vi "TRANCON-HARDWARE-SERVER.vi"() -> ()   [LabVIEW 2015]
doc: "MAIN vi for TRANCON project"
uses:
  dependecies/XControls/StartButton/StartButton.xctl
  <vilib>/NI/STM/Connection Manager/TCP/TCP Connection Method.ctl
  Classes/Control/Control-Server/Control-Server.lvclass
  dependecies/ControlsVIs/Clusters-def/DEFs_SERVER_buttons_refs.ctl
  Classes/Control/Control-Server/Control-Server.lvclass/Control-Server.ctl
  Classes/GeneralFunctionality/GeneralFunctionality.lvclass/GeneralFunctionality.ctl
  <vilib>/Platform/TimedLoop/XDataNode/timing_clust.ctl
  <vilib>/Platform/TimedLoop/XDataNode/nitl_modes.ctl
  <vilib>/Platform/TimedLoop/XDataNode/wakeup.ctl
  dependecies/ControlsVIs/Clusters-def/Message types.ctl
  dependecies/ControlsVIs/Clusters-def/SERVER-Commands.ctl
  Classes/Config/config_names_def.ctl
  <vilib>/NI/STM/TCP/Write Meta Data (TCP Ref).vi
  <vilib>/NI/STM/TCP/Write Meta Data (TCP Clst).vi
  <vilib>/Platform/TimedLoop/XDataNode/XDataNode.xnode
  Classes/Config/Config.lvclass
  <vilib>/NI/STM/NI STM.lvlib
  <vilib>/Platform/TimedLoop/XDataNode/XDNodeRunTimeDep.lvlib
  Classes/Message/Message.lvclass
  Classes/GeneralFunctionality/GeneralFunctionality.lvclass
panel:
  in  "DB Set":bool
  in  "DB connect":bool
  in  "OSc Set":bool
  in  "Oscilloscope connect":bool
  in  "DAQmx Set":bool
  in  "DAQmx connect":bool
  in  "DET Set":bool
  in  "Detector connect":bool
  in  "DL Set":bool
  in  "DL connect":bool
  in  "All connect":bool
  in  "Pump connect":bool
  out "# clients":i32
  out "stop":bool
  in  "StartButton":bool(xcontrol)
  out "error out":cluster{bool, i32, "source":string} {"?" format="%f"}
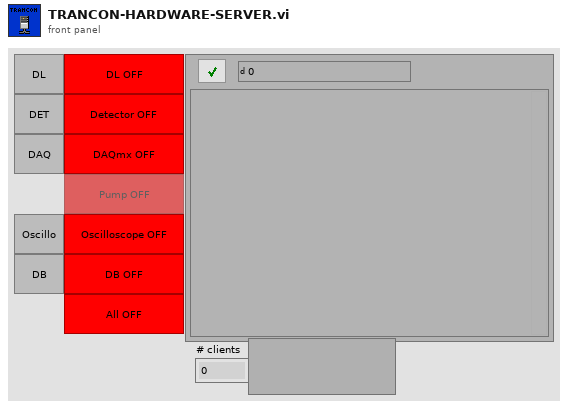
[diagram p1: front panel]
types:
  T1 = typedef "Control-Server.lvclass/DEFs_SERVER_buttons_refs.ctl" = cluster{"DL connect":refnum<vi>, "Detector connect":refnum<vi>, "DAQmx connect":refnum<vi>, "OSc connect":refnum<vi>, "DB connect":refnum<vi>, "All connect":refnum<vi>}
  T2 = typedef "NI STM.lvlib/TCP Connection Method.ctl" = enum16{"Initialize", "Add Connection", "Set Properties", "Get Connection(s)", "Remove Connection", "Remove All Connections", "Get Connection Count"}
  T3 = typedef "NI STM.lvlib/TCP Connection Info.ctl" = cluster{"connection ID":refnum<k5>, "meta data":T4[]}
  T4 = typedef "NI STM.lvlib/MetaDataElement.ctl" = string
  T5 = typedef "XDNodeRunTimeDep.lvlib/timing_clust.ctl" = cluster{"Expected End [f-1]":u64, "Actual End [f-1]":u64, "Finished Late? [f-1]":bool, "Expected End [i-1]":u64, "Actual End [i-1]":u64, "Finished Late? [i-1]":bool, "Expected Start [i]":u64, "Actual Start [i]":u64, "Expected Start [f]":u64, "Actual Start [f]":u64, "Source Name":string, "Structure Name":string, "Period":i64, "Deadline":i64, "Offset":i64, "Start":i64, "Priority":i32, "Timeout":i32, "Mode":T6, "Wakeup Reason":T7, "Error":errorcluster, "Source Type":string, "Secondary Source Type":string, "Global End Time":u64, "Global Start Time":u64, "Frame Duration":u64, "Iteration Duration":u64, "Assigned CPU":i32, "I/O Scan Engine Mode":u32}
  T6 = typedef "XDNodeRunTimeDep.lvlib/nitl_modes.ctl" = enum32{"No Change", "Process missed periods, maintain original phase", "Discard missed periods, maintain original phase", "Process missed periods, ignore original phase", "Discard missed periods, ignore original phase"}
  T7 = typedef "XDNodeRunTimeDep.lvlib/wakeup.ctl" = enum32{"Normal", "Aborted", "Asynchronous wakeup", "Timing source error", "Timed loop error", "Timeout"}
  T8 = typedef "Control-Server.lvclass/SERVER-Commands.ctl" = string
  T9 = typedef "Message types.ctl" = string
  T10 = typedef "Config.lvclass/config_names_def.ctl" = string
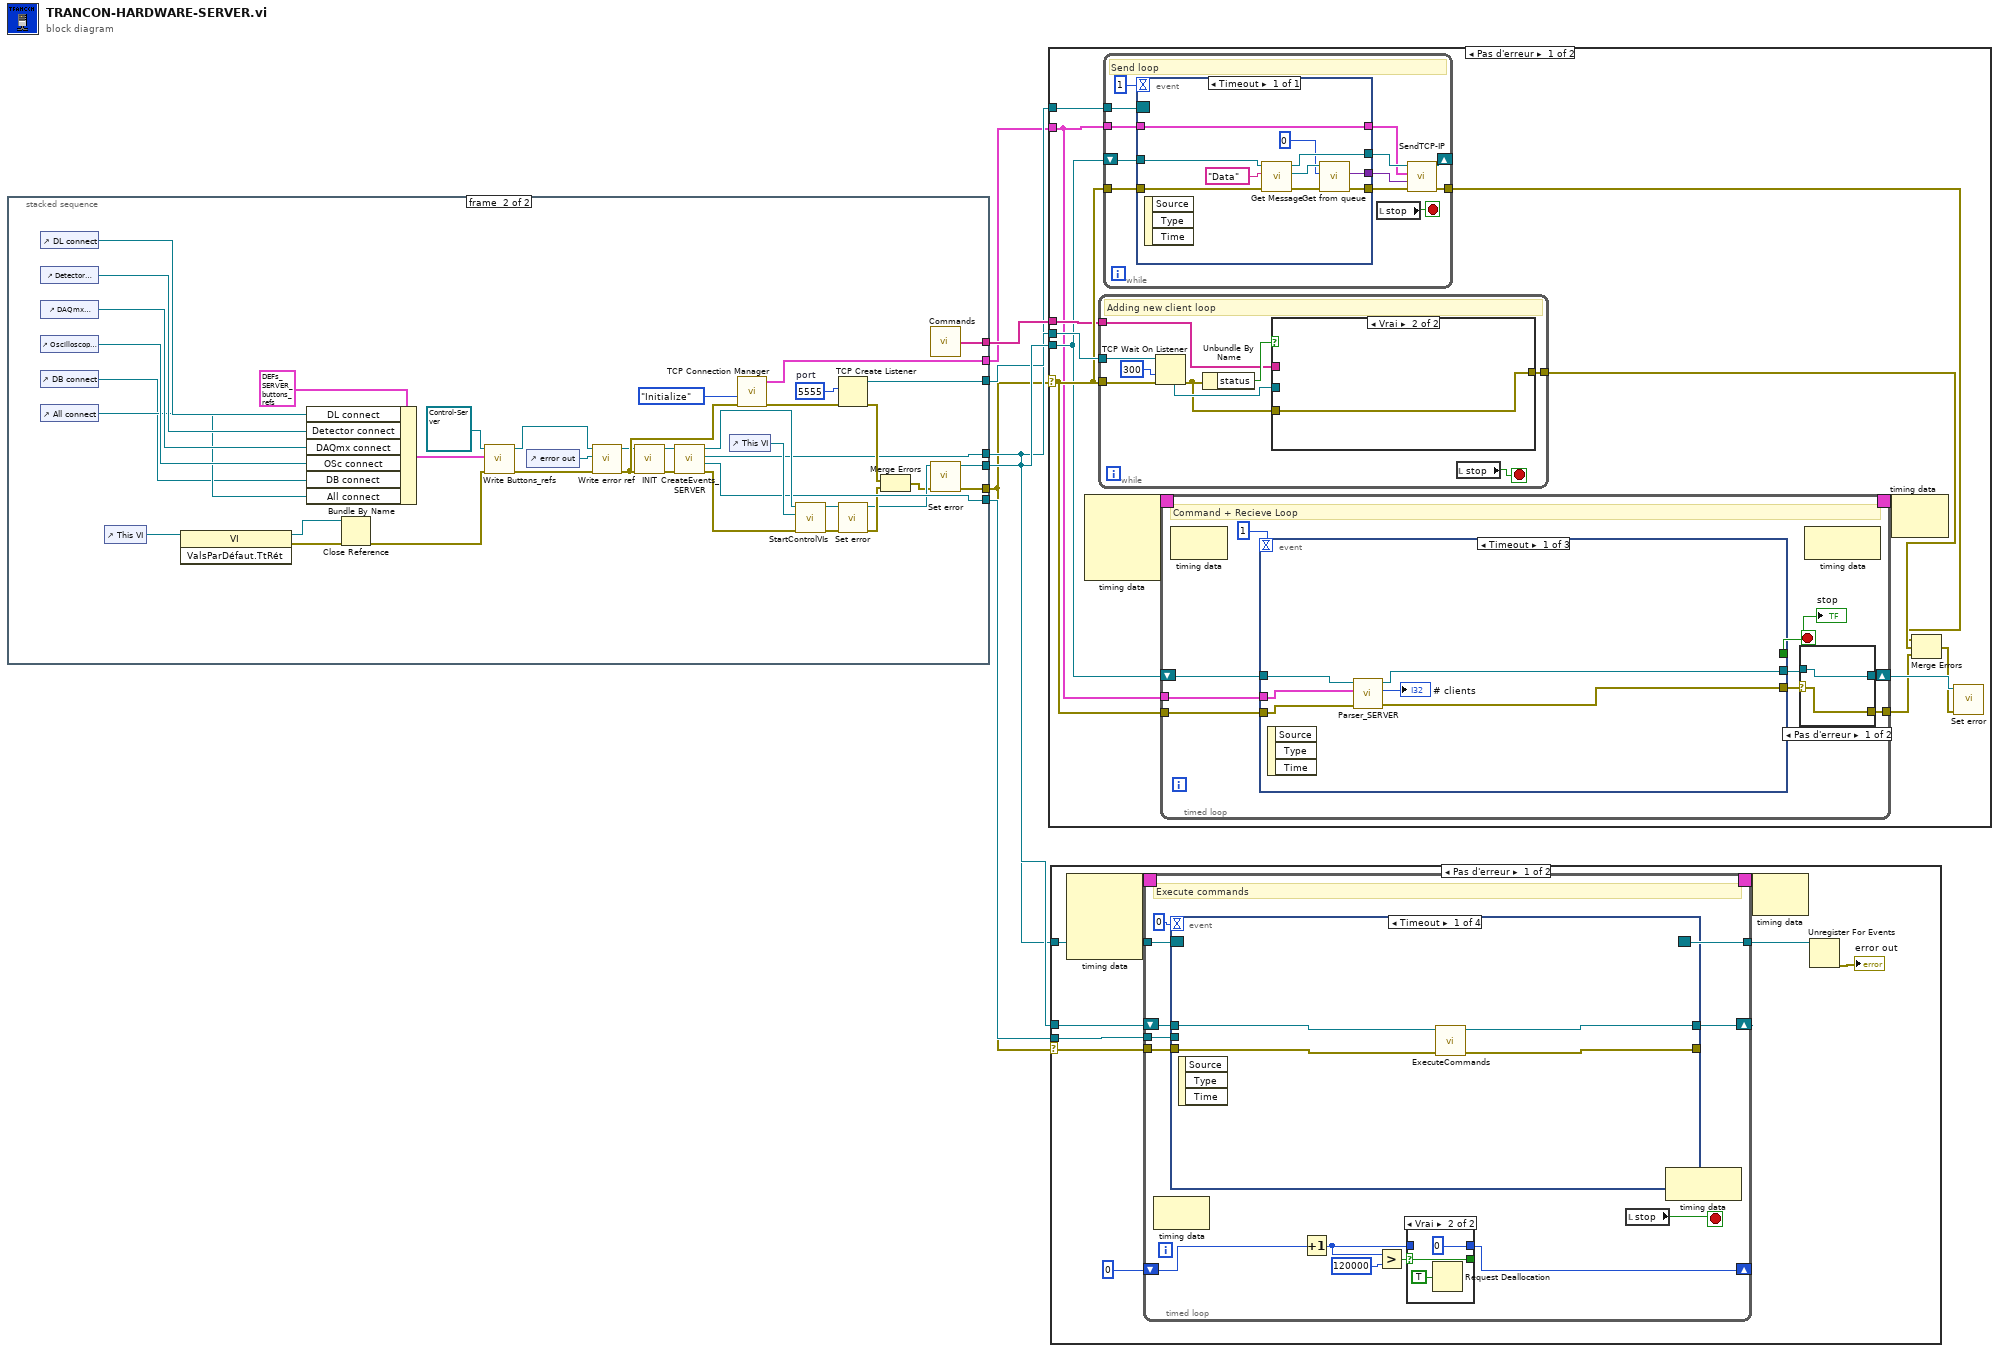
[diagram p0: block diagram]
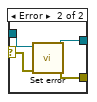
[diagram p2: hidden frame]
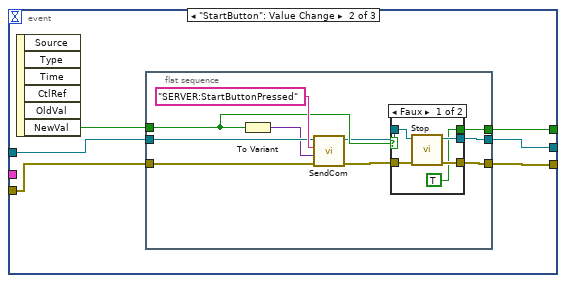
[diagram p3: hidden frame]
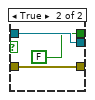
[diagram p4: hidden frame]
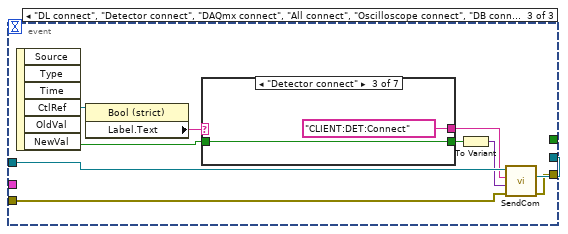
[diagram p5: hidden frame]
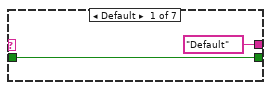
[diagram p6: hidden frame]
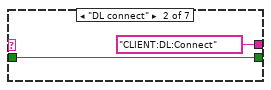
[diagram p7: hidden frame]
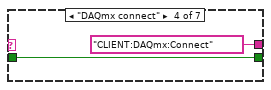
[diagram p8: hidden frame]
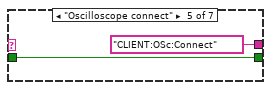
[diagram p9: hidden frame]
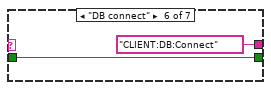
[diagram p10: hidden frame]
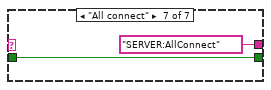
[diagram p11: hidden frame]
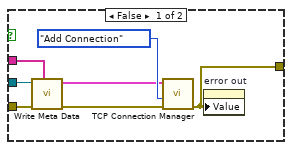
[diagram p12: hidden frame]
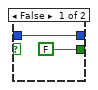
[diagram p14: hidden frame]
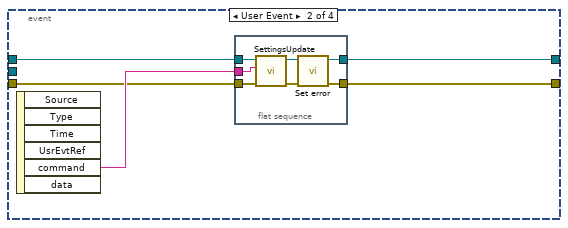
[diagram p15: hidden frame]
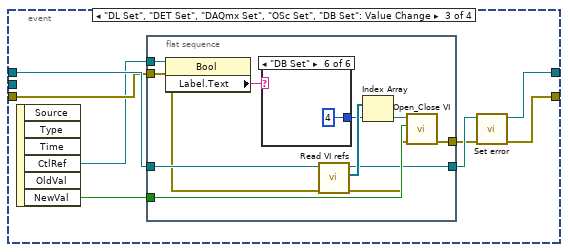
[diagram p16: hidden frame]
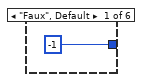
[diagram p17: hidden frame]
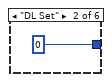
[diagram p18: hidden frame]
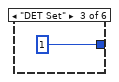
[diagram p19: hidden frame]
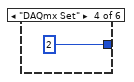
[diagram p20: hidden frame]
diagram:
  n1 = stacked-sequence {
    tunnel: [_ w24] -> w6
    tunnel: [_ w21] -> w3
    tunnel: [_ w42] -> w7
    tunnel: [_ w20] -> w5
    tunnel: [_ w35] -> w4
    tunnel: [_ w34] -> w1
    tunnel: [_ w23] -> w2
    frame #0 {
      n2 = flat-sequence {
        frame #0 {
        }
      }
    }
    frame #1 {
      w38 = u16 5555  # port
      n3 = control-ref of="DL connect"() -> (w15:refnum<vi>)
      n4 = control-ref of="Detector connect"() -> (w13:refnum<vi>)
      n5 = control-ref of="DAQmx connect"() -> (w12:refnum<vi>)
      n6 = control-ref of="Oscilloscope connect"() -> (w11:refnum<vi>)
      n7 = control-ref of="DB connect"() -> (w9:refnum<vi>)
      n8 = control-ref of="All connect"() -> (w10:refnum<vi>)
      n9 = control-ref of="This VI"() -> (w41:refnum<vi>)
      n10 = invoke class="VI" method="ValsParDéfaut.TtRét"(reference=w41) -> (reference out=w40:refnum<vi>, error out=w39:errorcluster)  [unwired: 2 in, 1 out]
      n11 = Bundle By Name(cluster=T1 {"DL connect"=refnum, "Detector connect"=refnum, "DAQmx connect"=refnum, "OSc connect"=refnum, "DB connect"=refnum, "All connect"=refnum} ("input cluster"), "DL connect"=w15, "Detector connect"=w13, "DAQmx connect"=w12, "OSc connect"=w11, "DB connect"=w9, "All connect"=w10) -> (w8:T1)
      n12 = Close Reference(reference=w40, error in (no error)=w39) -> (error out=w19:errorcluster)
      n13 = call "Write Buttons_refs.vi"("error in (no error)"=w19, "input cluster"=w8, "Control-Server in"=refnum<class "Control-Server.lvclass"> refnum) -> ("error out"=w18:errorcluster, "Control-Server out"=w17:refnum<class "Control-Server.lvclass">)  [unwired: 7 in]
      n14 = control-ref of="error out"() -> (w33:refnum<vi>)
      n15 = call "Write error ref.vi"("error in (no error)"=w18, "error"=w33, "GeneralFunctionality in"=w17) -> ("error out"=w29:errorcluster, "GeneralFunctionality out"=w28:refnum<class "Control-Server.lvclass">)  [unwired: 7 in]
      n16 = call-dynamic "INIT.vi"("error in (no error)"=w29, "Control-Server in"=w28) -> ("error out"=w32:errorcluster, "Control-Server out"=w45:refnum<class "Control-Server.lvclass">)  [unwired: 8 in]
      n17 = call "CreateEvents_SERVER.vi"("error in (no error)"=w32, "Control class"=w45) -> ("error out"=w43:errorcluster, "SettingsEventCom"=w42:refnum<user-event>, "Event Registration Refnum"=w21:refnum<event-registration>, "Control class out"=w44:refnum<class "Control-Server.lvclass">)  [unwired: 6 in]
      n18 = control-ref of="This VI"() -> (w46:refnum<vi>)
      n19 = call <vilib>:"TCP Connection Manager.vi"("error in"=w29, "method"=TCP_Connection_Method."Initialize") -> ("error out"=w36:errorcluster, "connection out"=w34:T3)  [unwired: 4 in, 4 out]
      n20 = call "StartControlVIs.vi"("entrée d'erreur (pas d'erreur)"=w43, "This VI"=w46, "Control in"=w44) -> ("sortie d'erreur"=w30:errorcluster, "Control out"=w31:refnum<class "Control-Server.lvclass">)  [unwired: 7 in]
      n21 = TCP Create Listener(8:w36, 10:w38) -> (0:w26:errorcluster, 3:w35:refnum<k5>)  [unwired: 3 in, 1 out]
      n22 = call "Set error.vi"("error in (no error)"=w30, "Control-Server in"=w31) -> ("error out"=w27:errorcluster, "Control-Server out"=w25:refnum<class "Control-Server.lvclass">)  [unwired: 8 in]
      n23 = Merge Errors(w26, w27) -> (w22:errorcluster)
      n24 = call "Commands.vi"() -> ("Commands"=w20:T4[])
      n25 = call "Set error.vi"("error in (no error)"=w22, "Control-Server in"=w25) -> ("error out"=w23:errorcluster, "Control-Server out"=w24:refnum<class "Control-Server.lvclass">)  [unwired: 8 in]
    }
  }
  n26 = case shown="Pas d'erreur" w2 {
    selector: w2 -> [w58 _]
    tunnel: w6 -> [w56 _]
    tunnel: w4 -> [w59 _]
    tunnel: w5 -> [w57 _]
    tunnel: w1 -> [w51 _]
    tunnel: w3 -> [w55 _]
    frame No Error {
      n27 = node-c288() -> (w54:T5)  [unwired: 4 in]
      n28 = while "Listen loop.  Append new connections to a synchronized queue." {
        tunnel: w57 -> [w161]
        tunnel: w58 -> [w159]
        tunnel: w59 -> [w158]
        tunnel: [w156] -> w49
        stop <- w157 stop-if-true
        # "Adding new client loop"
        n29 = TCP Wait On Listener(8:w159, 9:300 ("timeout ms (wait forever: -1)"), 11:w158) -> (0:w160:errorcluster, 4:w163:refnum<k5>)  [unwired: 1 in, 3 out]
        n30 = Unbundle By Name(w160) -> ("status"=w162:bool)
        n31 = case shown="Vrai" w162 {
          tunnel: w163 -> [w170 _]
          tunnel: w161 -> [w165 _]
          tunnel: w160 -> [w168 w171]
          tunnel: [w164 w171] -> w156
          frame False {
            n32 = call-poly <vilib>:"Write Meta Data.vi"("meta data"=w165, "error in"=w168, "connection ID"=w170) -> ("error out"=w169:errorcluster, "connection info out"=w166:T3)  [unwired: 7 in]
            n33 = call <vilib>:"TCP Connection Manager.vi"("error in"=w169, "method"=TCP_Connection_Method."Add Connection", "connection in"=w166) -> ("error out"=w164:errorcluster)  [unwired: 3 in, 5 out]
            n34 = property on="error out" class="Clust (strict)"("Value"=w164) -> ()  [unwired: 2 in, 2 out]
          }
          frame True {
          }
        }
        n35 = local read "stop"() -> (w157:bool)
      }
      n36 = while {
        tunnel: w58 -> [w143]
        tunnel: [w137] -> w48
        tunnel: w51 -> [w142]
        shift-right: [w136] -> _
        shift-left: w56 -> [w144]
        tunnel: w55 -> [w140]
        stop <- w133 stop-if-true
        # "Send loop"
        n37 = event shown="[0] Timeout" {
          selector: w140 -> [_]
          dyn-events: _ -> [_]
          timeout: 1 -> [_]
          tunnel: w144 -> [w154]
          tunnel: w143 -> [w153]
          tunnel: w142 -> [w149]
          tunnel: [w152] -> w139
          tunnel: [w151] -> w138
          tunnel: [w150] -> w135
          tunnel: [w149] -> w134
          event Timeout {
            n38 = event-data() -> ()  [unwired: 1 in, 3 out]
            n39 = call "Get Message.vi"("error in (no error)"=w153, "Message type"=T9 "Data", "GeneralFunctionality en entrée"=w154) -> ("error out"=w147:errorcluster, "Message.lvclass"=w146:refnum<class "Message.lvclass">, "GeneralFunctionality en sortie"=w150:refnum<class "Control-Server.lvclass">)  [unwired: 6 in]
            n40 = call "Get from queue.vi"("error in (no error)"=w147, "timeout in ms (-1)"=0, "Message in"=w146) -> ("error out"=w151:errorcluster, "Data"=w152:variant)  [unwired: 5 in, 2 out]
          }
        }
        n41 = local read "stop"() -> (w133:bool)
        n42 = call "SendTCP-IP.vi"("error in (no error)"=w138, "Data"=w139, "connection in"=w134, "Control in"=w135) -> ("error out"=w137:errorcluster, "Control out"=w136:refnum<class "Control-Server.lvclass">)  [unwired: 6 in]
      }
      n43 = timed-loop {
        tunnel: w58 -> [w68]
        tunnel: w51 -> [w67]
        shift-right: [w61] -> w52
        shift-left: w56 -> [w65]
        timing: w54 -> [_]
        timing-out: [_] -> w53
        tunnel: [w63] -> w50
        stop <- w64 stop-if-true
        # "Command + Recieve Loop"
        n44 = node-c288() -> ()  [unwired: 1 in, 1 out]
        n45 = event shown="[0] Timeout" {
          selector: _ -> [_ _ _]
          dyn-events: _ -> [_ _ _]
          timeout: 1 -> [_ _ _]
          tunnel: w65 -> [w78 w87 w115]
          tunnel: w68 -> [w82 w86 w116]
          tunnel: [w80 w83 w107] -> w60
          tunnel: w67 -> [w79 _ _]
          tunnel: [w77 w84 w108] -> w62
          tunnel: [_ w85 _] -> w64
          event Timeout {
            n46 = event-data() -> ()  [unwired: 1 in, 3 out]
            n47 = call "Parser_SERVER.vi"("error in (no error)"=w82, "connection in"=w79, "Control in"=w78) -> ("error out"=w80:errorcluster, "# clients"=→"# clients":i32, "Control out"=w77:refnum<class "Control-Server.lvclass">)  [unwired: 6 in]
          }
          event "StartButton": Value Change {
            n48 = event-data() -> ("NewVal"=w88:bool)  [unwired: 1 in, 5 out]
            n49 = flat-sequence {
              tunnel: w88 -> [w94]
              tunnel: w87 -> [w97]
              tunnel: [w91] -> w84
              tunnel: [w90] -> w83
              tunnel: w86 -> [w96]
              tunnel: [w89] -> w85
              frame #0 {
                n50 = To Variant(anything=w94) -> (Variant=w95:variant)
                n51 = call "SendCom.vi"("error in (no error)"=w96, "data"=w95, "Command"="SERVER:StartButtonPressed", "Control in"=w97) -> ("error out"=w92:errorcluster, "Control out"=w93:refnum<class "Control-Server.lvclass">)  [unwired: 6 in]
                n52 = case shown="Faux" w94 {
                  tunnel: [w103 w106] -> w91
                  tunnel: [w102 w105] -> w90
                  tunnel: w93 -> [w100 w106]
                  tunnel: w92 -> [w101 w105]
                  tunnel: [TRUE FALSE] -> w89
                  frame False {
                    n53 = call-dynamic "Stop.vi"("error in (no error)"=w101, "Control in"=w100) -> ("error out"=w102:errorcluster, "Control out"=w103:refnum<class "Control-Server.lvclass">)  [unwired: 8 in]
                  }
                  frame True {
                  }
                }
              }
            }
          }
          event "DL connect", "Detector connect", "DAQmx connect", "All connect", "Oscilloscope connect", "DB connect": Value Change {
            n54 = event-data() -> ("CtlRef"=w114:refnum<vi>, "NewVal"=w111:bool)  [unwired: 1 in, 4 out]
            n55 = property class="Bool (strict)"(reference=w114) -> ("Label.Text"=w113:string)  [unwired: 1 in, 2 out]
            n56 = case shown="\"Detector connect\"" w113 {
              tunnel: [T8 "Default" ("Commands") T8 "CLIENT:DL:Connect" ("Commands") T8 "CLIENT:DET:Connect" ("Commands") T8 "CLIENT:DAQmx:Connect" ("Commands") T8 "CLIENT:OSc:Connect" ("Commands") T8 "CLIENT:DB:Connect" ("Commands") T8 "SERVER:AllConnect" ("Commands")] -> w112
              tunnel: w111 -> [w117 w119 w121 w123 w125 w127 w129]
              tunnel: [w117 w119 w121 w123 w125 w127 w129] -> w110
              frame Default {
              }
              frame "DL connect" {
              }
              frame "Detector connect" {
              }
              frame "DAQmx connect" {
              }
              frame "Oscilloscope connect" {
              }
              frame "DB connect" {
              }
              frame "All connect" {
              }
            }
            n57 = To Variant(anything=w110) -> (Variant=w109:variant)
            n58 = call "SendCom.vi"("error in (no error)"=w116, "data"=w109, "Command"=w112, "Control in"=w115) -> ("error out"=w107:errorcluster, "Control out"=w108:refnum<class "Control-Server.lvclass">)  [unwired: 6 in]
          }
        }
        "stop" <- w64
        n59 = case shown="Pas d'erreur" w60 {
          selector: w60 -> [w69 w71]
          tunnel: [w69 w74] -> w63
          tunnel: w62 -> [w70 w73]
          tunnel: [w70 w72] -> w61
          frame No Error {
          }
          frame Error {
            n60 = call "Set error.vi"("error in (no error)"=w71, "Control-Server in"=w73) -> ("error out"=w74:errorcluster, "Control-Server out"=w72:refnum<class "Control-Server.lvclass">)  [unwired: 8 in]
          }
        }
        n61 = node-c288() -> ()  [unwired: 1 in, 1 out]
      }
      n62 = node-c288(w53) -> ()  [unwired: 1 out]
      n63 = Merge Errors(w48, w49, w50) -> (w47:errorcluster)
      n64 = call "Set error.vi"("error in (no error)"=w47, "Control-Server in"=w52) -> ()  [unwired: 8 in, 2 out]
    }
    frame Error {
    }
  }
  n65 = case shown="Pas d'erreur" w2 {
    selector: w2 -> [w178 _]
    tunnel: w6 -> [w180 _]
    tunnel: w3 -> [w177 _]
    tunnel: w7 -> [w176 _]
    frame No Error {
      n66 = node-c288() -> (w175:T5)  [unwired: 4 in]
      n67 = timed-loop {
        shift-right: [w191] -> _
        shift-left: w180 -> [w192]
        tunnel: w178 -> [w193]
        tunnel: [w190] -> w179
        tunnel: w177 -> [w189]
        tunnel: w176 -> [w188]
        timing: w175 -> [_]
        timing-out: [_] -> w174
        shift-right: [w181] -> _
        shift-left: 0 -> [w182]
        stop <- w186 stop-if-true
        # "Execute commands"
        n68 = node-c288() -> ()  [unwired: 1 in, 1 out]
        n69 = event shown="[0] Timeout" {
          selector: w189 -> [_ _ _ _]
          dyn-events: [_ _ _ _] -> w190
          timeout: 0 -> [_ _ _ _]
          tunnel: [w201 w205 w219 w242] -> _
          tunnel: w193 -> [w203 w207 w223 w247]
          tunnel: w192 -> [w204 w208 w224 w244]
          tunnel: [w202 w206 w218 w243] -> w191
          tunnel: w188 -> [_ _ _ w246]
          event Timeout {
            n70 = event-data() -> ()  [unwired: 1 in, 3 out]
            n71 = call "ExecuteCommands.vi"("error in (no error)"=w203, "Control in"=w204) -> ("error out"=w201:errorcluster, "Control out"=w202:refnum<class "Control-Server.lvclass">)  [unwired: 8 in]
          }
          event User Event {
            n72 = event-data() -> ("command"=w209:string)  [unwired: 1 in, 5 out]
            n73 = flat-sequence {
              tunnel: w209 -> [w216]
              tunnel: w208 -> [w215]
              tunnel: w207 -> [w214]
              tunnel: [w212] -> w206
              tunnel: [w210] -> w205
              frame #0 {
                n74 = call "SettingsUpdate.vi"("error in (no error)"=w214, "Command"=w216, "Control in"=w215) -> ("error out"=w211:errorcluster, "Control out"=w213:refnum<class "Control-Server.lvclass">)  [unwired: 7 in]
                n75 = call "Set error.vi"("error in (no error)"=w211, "Control-Server in"=w213) -> ("error out"=w210:errorcluster, "Control-Server out"=w212:refnum<class "Control-Server.lvclass">)  [unwired: 8 in]
              }
            }
          }
          event "DL Set", "DET Set", "DAQmx Set", "OSc Set", "DB Set": Value Change {
            n76 = event-data() -> ("CtlRef"=w217:refnum<vi>, "NewVal"=w222:bool)  [unwired: 1 in, 4 out]
            n77 = flat-sequence {
              tunnel: [w230] -> w221
              tunnel: w224 -> [w233]
              tunnel: w223 -> [w226]
              tunnel: w222 -> [w235]
              tunnel: [w234] -> w220
              tunnel: w217 -> [w229]
              frame #0 {
                n78 = property class="Bool"(reference=w229) -> ("Label.Text"=w228:string)  [unwired: 1 in, 2 out]
                n79 = case shown="\"DB Set\"" w228 {
                  tunnel: [-1 0 1 2 3 4] -> w227
                  frame "Faux", Default {
                  }
                  frame "DL Set" {
                  }
                  frame "DET Set" {
                  }
                  frame "DAQmx Set" {
                  }
                  frame "OSc Set" {
                  }
                  frame "DB Set" {
                  }
                }
                n80 = call-dynamic "Read VI refs.vi"("error in (no error)"=w226, "Control in"=w233) -> ("error out"=w225:errorcluster, "VI refs"=w232:refnum<vi>[], "Control out"=w230:refnum<class "Control-Server.lvclass">)  [unwired: 7 in]
                n81 = Index Array(array=w232, index=w227) -> (element=w231:refnum<vi>)
                n82 = call "Open_Close VI.vi"("error in (no error)"=w225, "NewVal"=w235, "VI in"=w231) -> ("error out"=w234:errorcluster)  [unwired: 8 in]
              }
            }
            n83 = call "Set error.vi"("error in (no error)"=w220, "Control-Server in"=w221) -> ("error out"=w219:errorcluster, "Control-Server out"=w218:refnum<class "Control-Server.lvclass">)  [unwired: 8 in]
          }
          event Menu Selection (User) {
            n84 = event-data() -> ("ItemTag"=w248:string)  [unwired: 1 in, 6 out]
            n85 = flat-sequence {
              tunnel: w248 -> [w254]
              tunnel: w247 -> [w253]
              tunnel: [w252] -> w245
              tunnel: w244 -> [w251]
              tunnel: w246 -> [w249]
              frame #0 {
                n86 = case shown="\"Settings\"" w254 {
                  tunnel: w253 -> [w258 w263]
                  tunnel: [w261 w263] -> w252
                  tunnel: w251 -> [w260 _]
                  tunnel: TRUE ("stop? (T)") -> [_ w262]
                  tunnel: w249 -> [w256 _]
                  frame "Settings" {
                    n87 = call "Read Configuration dict.vi"("error in (no error)"=w258, "Config Name"=T10 "MainConfig" ("Combo Box"), "Control in"=w260) -> ("error out"=w255:errorcluster, "Config"=w257:refnum<class "Config.lvclass">)  [unwired: 6 in, 1 out]
                    n88 = call "SettingsVI_RUN.vi"("error in (no error)"=w255, "user event"=w256, "Config in"=w257) -> ("error out"=w261:errorcluster)  [unwired: 7 in, 1 out]
                  }
                  frame "Exit", Default {
                    n89 = Stop(stop? (T)=w262) -> ()
                  }
                }
              }
            }
            n90 = call "Set error.vi"("error in (no error)"=w245, "Control-Server in"=w244) -> ("error out"=w242:errorcluster, "Control-Server out"=w243:refnum<class "Control-Server.lvclass">)  [unwired: 8 in]
          }
        }
        n91 = Increment(x=w182) -> (x+1=w183:i32)
        n92 = Greater?(x=w183, y=120000) -> (0:w184:bool)
        n93 = case shown="Vrai" w184 {
          selector: w184 -> [_ w198]
          tunnel: [FALSE w198] -> _
          tunnel: [w194 0] -> w181
          tunnel: w183 -> [w194 _]
          frame False {
          }
          frame True {
            n94 = Request Deallocation(TRUE ("flag")) -> ()
          }
        }
        n95 = local read "stop"() -> (w186:bool)
        n96 = node-c288() -> ()  [unwired: 1 in, 1 out]
      }
      n97 = node-c288(w174) -> ()  [unwired: 1 out]
      n98 = Unregister For Events(event registration refnum=w179) -> (error out=→"error out":errorcluster)  [unwired: 1 in]
    }
    frame Error {
    }
  }
